vi "Read.vi"(8 "error in (no error)":errorcluster, 9 "timeout ms (25000)":i32, 10 "# bytes to read":i32, 11 "VISA TCP in":refnum<class "VISA TCP.lvclass">) -> (0 "error out":errorcluster, 1 "timed out?":bool, 2 "Read Bytes":u8[](array[numeric]), 3 "VISA TCP out":refnum<class "VISA TCP.lvclass">)   [LabVIEW 2021, in "Sockets.lvlib" / "VISA TCP.lvclass"]
doc: "Reads data from a socket connection.\nWebSockets 2.0.1.40\nSam Sharp - MediaMongrels Ltd\nCopyright (c) 2019, MediaMongrels Ltd"
uses:
  VISA TCP.lvclass
  VISA TCP.lvclass/VISA TCP.ctl
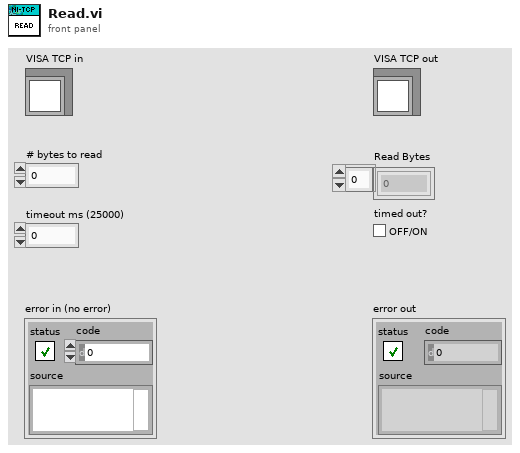
[diagram p1: front panel]
types:
  T1 = enum16{"Standard", "Buffered", "CRLF", "Immediate"}
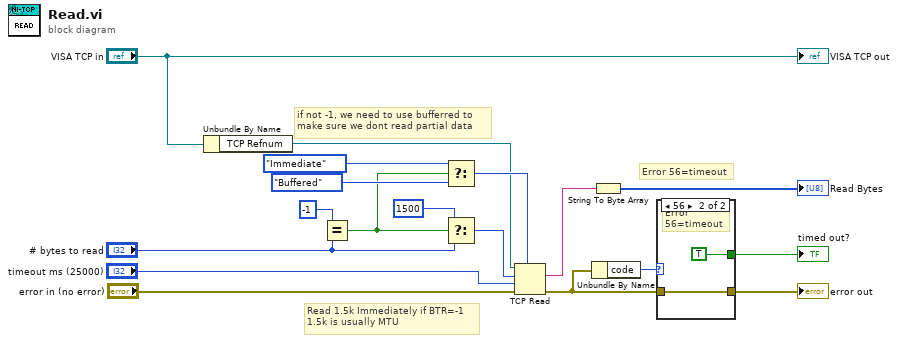
[diagram p0: block diagram]
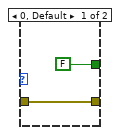
[diagram p2: hidden frame]
diagram:
  # "Error 56=timeout"
  # "Read 1.5k Immediately if BTR=-1\n1.5k is usually MTU"
  # "if not -1, we need to use bufferred to\nmake sure we dont read partial data"
  n1 = Unbundle By Name("VISA TCP in") -> ("TCP Refnum"=w7:refnum<k5>)
  n2 = Equal?(x=-1, y="# bytes to read") -> (x = y?=w13:bool)
  n3 = Select(t=T1."Immediate" ("mode (standard)"), s=w13, f=T1."Buffered" ("mode (standard)")) -> (s? t:f=w14:T1)
  n4 = Select(t=1500, s=w13, f="# bytes to read") -> (s? t:f=w12:i32)
  n5 = TCP Read(connection ID=w7, bytes to read=w12, error in (no error)="error in (no error)", 7:w14, 9:"timeout ms (25000)") -> (data out=w9:string, error out=w10:errorcluster)  [unwired: 1 out]
  n6 = Unbundle By Name(w10) -> ("code"=w8:i32)
  n7 = String To Byte Array(string=w9) -> (unsigned byte array=→"Read Bytes":u8[])
  n8 = case shown="56" w8 {
    tunnel: w10 -> [w20 w21]
    tunnel: [w20 w21] -> w3
    tunnel: [FALSE TRUE] -> w1
    frame 0, Default {
    }
    frame 56 {
      # "Error 56=timeout"
    }
  }
  "error out" <- w3
  "timed out?" <- w1
  "VISA TCP out" <- "VISA TCP in"
